vi "Guia1_2.vi"() -> ()   [LabVIEW 2016]
panel:
  out "Numeric 6":i32
  out "Boolean 4":bool
  out "String 3":string
  out "Numeric 5":i32
  in  "Numeric 4":dbl
  out "Boolean 2":bool
  in  "Boolean":bool
  in  "String 2":string
  out "String":string
  out "Numeric 3":i32
  out "Numeric 2":dbl
  in  "Numeric":i32
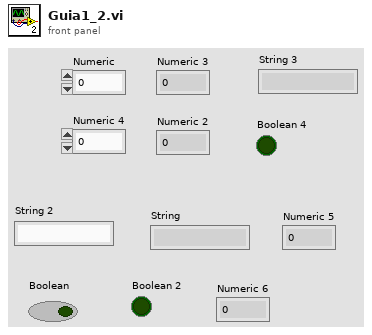
[diagram p1: front panel]
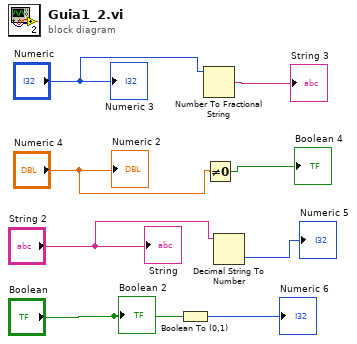
[diagram p0: block diagram]
diagram:
  n1 = Boolean To (0,1)(Boolean="Boolean") -> (0, 1=→"Numeric 6":i16)
  n2 = Number To Fractional String(number="Numeric") -> (F-format string=→"String 3":string)  [unwired: 3 in]
  n3 = Not Equal To 0?(x="Numeric 4") -> (x != 0?=→"Boolean 4":bool)
  n4 = Decimal String To Number(string="String 2") -> (number=→"Numeric 5":i32)  [unwired: 2 in, 1 out]
  "Numeric 2" <- "Numeric 4"
  "Numeric 3" <- "Numeric"
  "String" <- "String 2"
  "Boolean 2" <- "Boolean"
